vi "Test Math.vi"() -> ()   [LabVIEW 2021]
uses:
  Source/Constants/Support/DBL/Const_DBL.lvclass
  C:/TSA/LV_Abstract/Source/Abs_Types/Double Float/Abs_Double Float.lvclass
  Source/Abs_Types/I32 Integer/Abs_I32 Integer.lvclass
  C:/Program Files (x86)/National Instruments/LabVIEW 2021/vi.lib/TSA/Abstract Data Classes/Abs_Types/Numeric/Abs_Numeric.lvclass
  Source/Constants/Support/DBL/DBL.vi
  Source/Constants/Support/I32/I32.vi
  Source/Functions/Math/Support/Subtract/I32/Method_Const.vi
  Source/Functions/Math/Support/Add/DBL/Method.vi
  Source/Functions/Math/Support/Multiply/DBL/Method_Const.vi
  Source/Abs_Types/Double Float/Abs_Double Float.lvclass
  Source/Functions/Math/Support/Add/DBL/Add_DBL.lvclass
  Source/Constants/Support/I32/Const_I32.lvclass
  Source/Functions/Math/Support/Subtract/I32/Subtract_I32.lvclass
  Source/Functions/Math/Support/Multiply/DBL/Multiply_DBL.lvclass
  C:/TSA/LV_Abstract/Source/Abs_Types/Integer/Abs_Integer.lvclass
  C:/Program Files (x86)/National Instruments/LabVIEW 2021/vi.lib/TSA/Abstract Data Classes/Abs_Types/Value/Abs_Value.lvclass
  C:/Program Files (x86)/National Instruments/LabVIEW 2021/vi.lib/TSA/Abstract Data Classes/Abs_Types/Type/Abs_Type.lvclass
  C:/TSA/LV_Abstract/Source/Abs_Types/I32 Integer/Abs_I32 Integer.lvclass
  C:/TSA/LV_Abstract/Source/Abs_Types/Floating Point/Abs_Floating Point.lvclass
  C:/TSA/LV_Abstract/Source/Constants/Support/DBL/Const_DBL.lvclass
panel:
  in  "Numeric 5":dbl
  in  "Numeric 4":dbl
  in  "Numeric 3":i32
  in  "Numeric 2":dbl
  out "Numeric":dbl
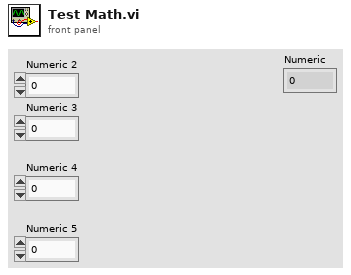
[diagram p1: front panel]
types:
  T1 = typedef "Subtract_I32.lvclass/Abs Type.ctl" = refnum<class "Abs_I32 Integer.lvclass">
  T2 = typedef "Abs_Double Float.lvclass/Type.ctl" = dbl
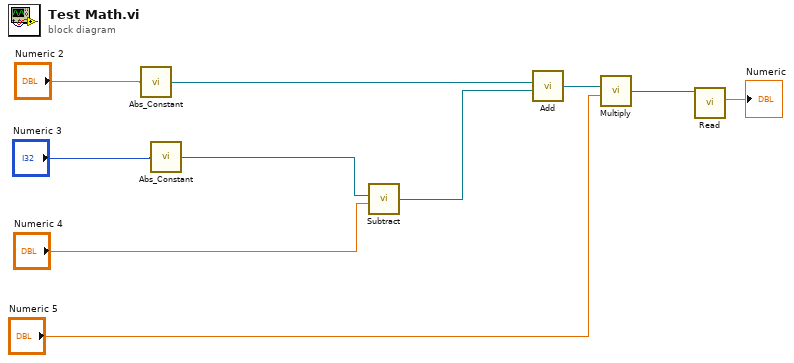
[diagram p0: block diagram]
diagram:
  n1 = call-poly "Abs_Constant.vi"("Value"="Numeric 2") -> ("Constant"=w5:refnum<class "Const_DBL.lvclass">)  [unwired: 4 in]
  n2 = call-poly "Abs_Constant.vi"("Value"="Numeric 3") -> ("Constant"=w6:refnum<class "Abs_I32 Integer.lvclass">)  [unwired: 4 in]
  n3 = call-poly "Subtract.vi"("Value"="Numeric 4", "Input A"=w6) -> ("Result"=w4:T1)  [unwired: 4 in]
  n4 = call-poly "Add.vi"("Abs_Types.lvlib:Numeric.lvclass"=w4, "Input A"=w5) -> ("Result"=w3:refnum<class "Abs_Double Float.lvclass">)  [unwired: 4 in]
  n5 = call-poly "Multiply.vi"("Value"="Numeric 5", "Input A"=w3) -> ("Result"=w10:refnum<class "Abs_Double Float.lvclass">)  [unwired: 4 in]
  n6 = call-dynamic "Read.vi"("Double Float.lvclass_340760 in"=w10) -> ("Value"=→"Numeric":T2)  [unwired: 8 in, 2 out]
